vi "4112_Current _Chan Config Dialog_RTM.vi"(8 "error in (no error)":errorcluster, 11 "CD PTR":T1 format="%.0x") -> (0 "error out":errorcluster, 1 "Channels to Add":u16[](array[numeric]), 2 "Voltage Limit (out)":dbl, 3 "Initial Current Value (out)":dbl, 5 "Cancel (out)":bool)   [LabVIEW 2018, in "NI PXI-4110 Programmable Power Supply Custom Device.lvlib"]
doc: "This VI is used to collect all the desired confifugurations for new 4112 Voltage Channels. Note: A true on Sense Mode = Remote and a False = Local."
uses:
  NI PXI-4110 Programmable Power Supply Custom Device.lvlib
  <vilib>/NI Veristand/Custom Device API/Custom Device Item Ref.ctl
  Power_Supply_In_Use.ctl
  4110_Global.vi
  <vilib>/NI Veristand/Custom Device API/Get Item Property (U16).vi
  <vilib>/NI Veristand/Custom Device API/Get Item Property (Boolean).vi
  <vilib>/NI VeriStand/Custom Device API/Custom Device API.lvlib
panel:
  in  "Channel(s) to add":cluster{"Channel 0":bool, "Channel 1":bool}
  in  "Cancel":bool
  in  "OK Button":bool
  in  "Initial Current Value":dbl format="%.4f"
  in  "Voltage Limit":dbl
  # "Current Channels"
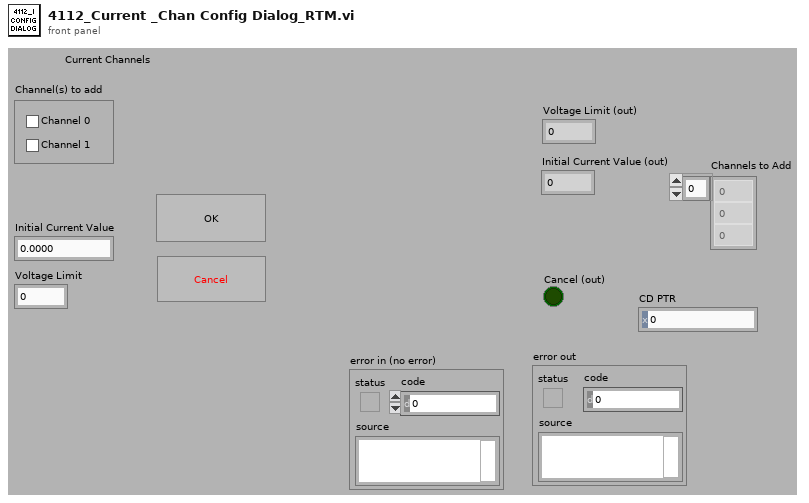
[diagram p1: front panel]
types:
  T1 = typedef "Custom Device API.lvlib/Custom Device Item Ref.ctl" = u64
  T2 = enum8{"Enabled", "Disabled", "Disabled and Grayed Out"}
  T3 = typedef "Custom Device API.lvlib/Custom Device Item Info.ctl" = cluster{"Name":string, "Is Channel":bool, "GUID":string, "Is Waveform":bool}
  T4 = typedef "NI PXI-4110 Programmable Power Supply Custom Device.lvlib/Power_Supply_In_Use.ctl" = enum16{"PXIe-4112", "PXI-4110"}
  T5 = cluster{"V_min":dbl, "V_max":dbl, "I_min":dbl, "I_max":dbl}
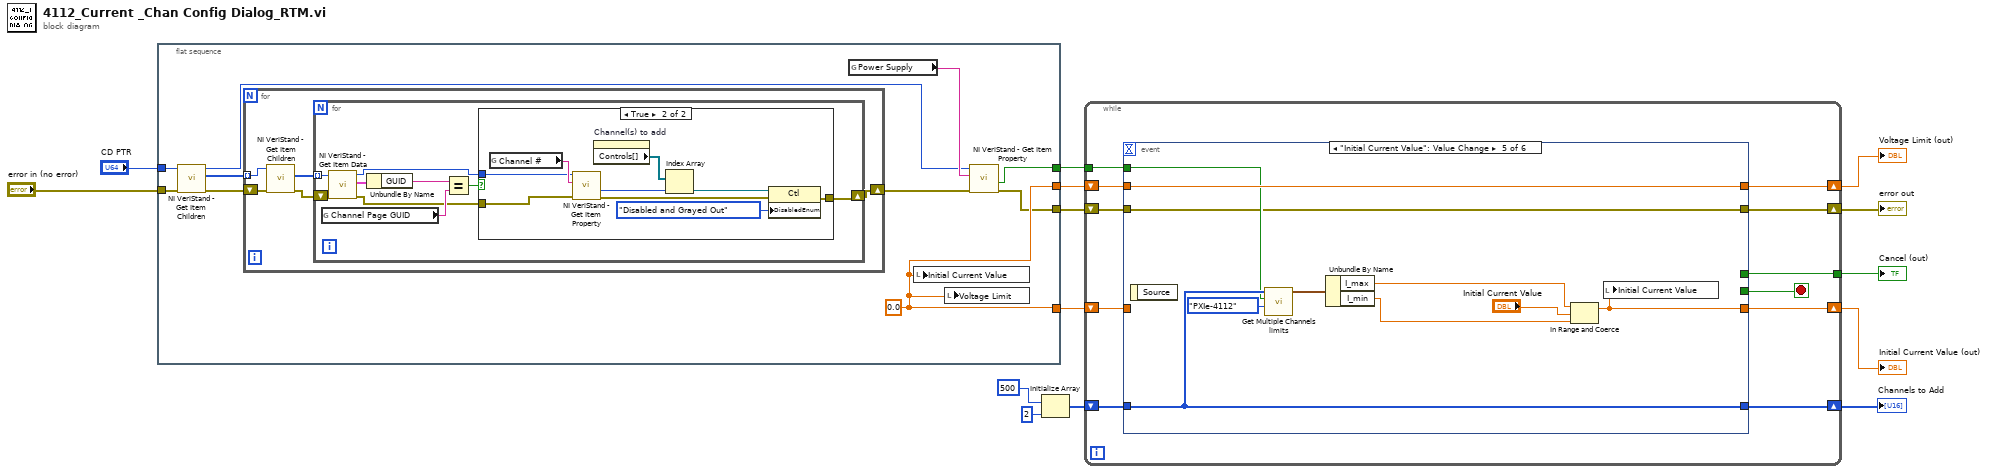
[diagram p0: block diagram]
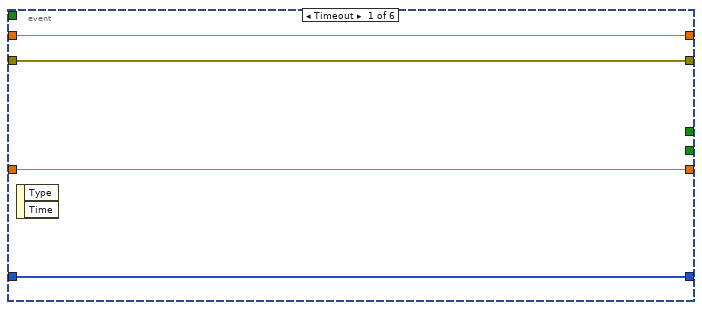
[diagram p3: hidden frame]
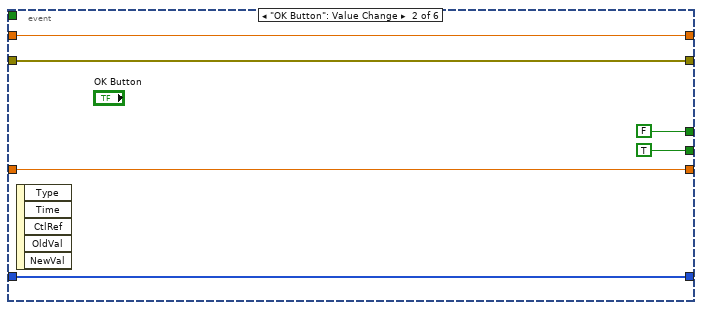
[diagram p4: hidden frame]
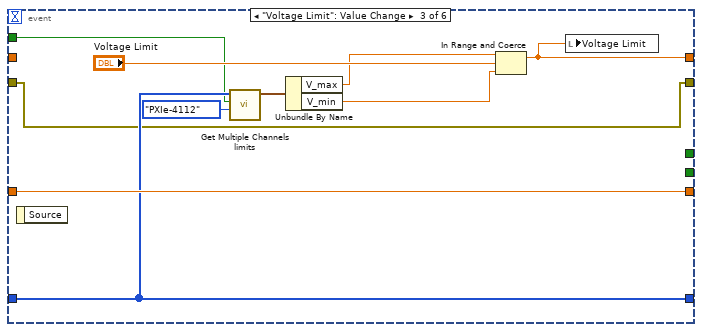
[diagram p5: hidden frame]
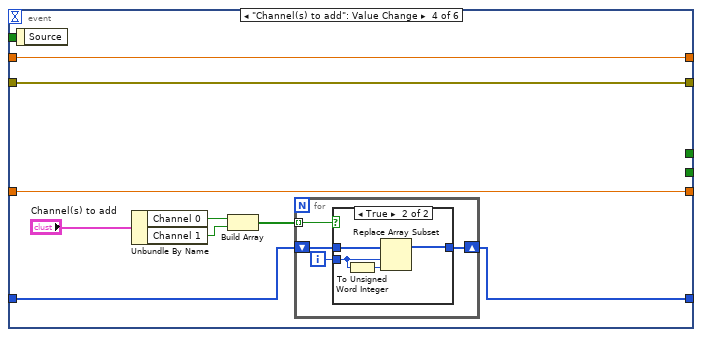
[diagram p6: hidden frame]
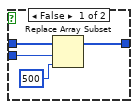
[diagram p7: hidden frame]
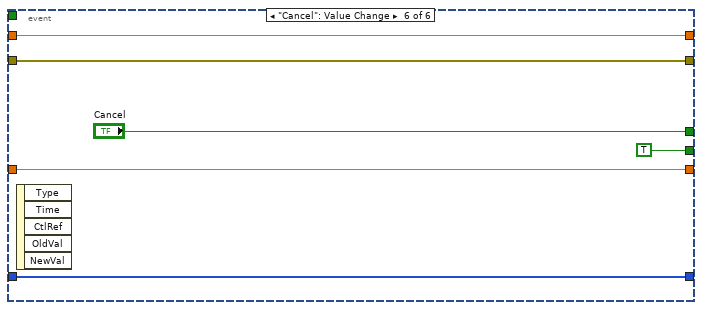
[diagram p8: hidden frame]
diagram:
  n1 = flat-sequence {
    tunnel: [w16] -> w14
    tunnel: [w20] -> w9
    tunnel: [w20] -> w8
    tunnel: "error in (no error)" -> [w24]
    tunnel: "CD PTR" -> [w23]
    tunnel: [w17] -> w5
    frame #0 {
      w20 = 0.0
      n2 = call <vilib>:"NI VeriStand - Get Item Children.vi"("error in (no error)"=w24, "Item Ref in"=w23) -> ("error out"=w21:errorcluster, "Child Refs"=w22:T1[], "Item Ref out"=w15:T1)  [unwired: 6 in, 1 out]
      n3 = for {
        tunnel: w22 -> [w28] mode=indexing
        shift-right: [w29] -> w19
        shift-left: w21 -> [w27]
        n4 = call <vilib>:"NI VeriStand - Get Item Children.vi"("error in (no error)"=w27, "Item Ref in"=w28) -> ("error out"=w25:errorcluster, "Child Refs"=w26:T1[])  [unwired: 6 in, 2 out]
        n5 = for {
          tunnel: w26 -> [w31] mode=indexing
          shift-right: [w38] -> w29
          shift-left: w25 -> [w30]
          n6 = global read "4110_Global.vi" "Channel Page GUID"() -> (w35:string)
          n7 = call <vilib>:"NI VeriStand - Get Item Data.vi"("error in (no error)"=w30, "Item Ref in"=w31) -> ("error out"=w33:errorcluster, "Item Info"=w37:T3, "Item Ref out"=w34:T1)  [unwired: 6 in, 1 out]
          n8 = Unbundle By Name(w37) -> ("GUID"=w36:string)
          n9 = Equal?(x=w36, y=w35) -> (x = y?=w32:bool)
          n10 = case shown="True" w32 {
            tunnel: [w39 w42] -> w38
            tunnel: w34 -> [_ w41]
            tunnel: w33 -> [w39 w40]
            frame False {
            }
            frame True {
              n11 = global read "4110_Global.vi" "Channel #"() -> (w48:string)
              n12 = call-poly <vilib>:"NI VeriStand - Get Item Property.vi"("error in (no error)"=w40, "Property Name"=w48, "Item Ref in"=w41) -> ("error out"=w43:errorcluster, "Value"=w44:u16)  [unwired: 5 in, 2 out]
              n13 = property on="Channel(s) to add" class="Clust (strict)"() -> ("Controls[]"=w46:refnum<vi>[])  [unwired: 2 in, 2 out]
              n14 = Index Array(array=w46, index=w44) -> (element=w47:refnum<vi>)
              n15 = property class="Ctl"(reference=w47, error in=w43, "DisabledEnum"=T2."Disabled and Grayed Out" ("Disabled")) -> (error out=w42:errorcluster)  [unwired: 1 out]
            }
          }
        }
      }
      n16 = global read "4110_Global.vi" "Power Supply"() -> (w18:string)
      n17 = local write "Initial Current Value"(w20) -> ()
      n18 = local write "Voltage Limit"(w20) -> ()
      n19 = call-poly <vilib>:"NI VeriStand - Get Item Property.vi"("error in (no error)"=w19, "Property Name"=w18, "Item Ref in"=w15) -> ("error out"=w16:errorcluster, "Value"=w17:bool)  [unwired: 5 in, 2 out]
    }
  }
  n20 = Initialize Array(u16 500 ("element"), 2 ("dimension size")) -> (w2:u16[])
  n21 = while {
    tunnel: [w55] -> w10
    shift-right: [w58] -> w13
    shift-left: w14 -> [w59]
    shift-right: [w57] -> w12
    shift-left: w9 -> [w53]
    shift-right: [w56] -> w11
    shift-left: w8 -> [w52]
    tunnel: w5 -> [w51]
    shift-right: [w49] -> w1
    shift-left: w2 -> [w50]
    stop <- w54 stop-if-true
    n22 = event shown="[4] \"Initial Current Value\": Value Change" {
      selector: _ -> [_ _ _ _ _ _]
      dyn-events: _ -> [_ _ _ _ _ _]
      timeout: _ -> [_ _ _ _ _ _]
      tunnel: [w63 w66 w79 w88 w109 w114] -> w57
      tunnel: [w62 w65 w77 w87 w108 w113] -> w56
      tunnel: w59 -> [w60 w69 w70 w80 w101 w111]
      tunnel: [w60 w69 w70 w80 w101 w111] -> w58
      tunnel: [_ FALSE ("Cancel") _ _ _ "Cancel"] -> w55
      tunnel: [_ TRUE ("Cancel") _ _ _ TRUE ("Cancel")] -> w54
      tunnel: w53 -> [w63 w66 w79 w88 _ w114]
      tunnel: w52 -> [w62 w65 _ w87 w108 w113]
      tunnel: w51 -> [_ _ w75 _ w106 _]
      tunnel: w50 -> [w61 w64 w76 w82 w107 w112]
      tunnel: [w61 w64 w76 w81 w107 w112] -> w49
      event Timeout {
        n23 = event-data() -> ()  [unwired: 1 in, 2 out]
      }
      event "OK Button": Value Change {
        n24 = event-data() -> ()  [unwired: 1 in, 5 out]
      }
      event "Voltage Limit": Value Change {
        n25 = event-data() -> ()  [unwired: 1 in, 1 out]
        n26 = call "Get Multiple Channels limits.vi"("Power Supply In Use"=Power_Supply_In_Use."PXIe-4112", "External Supply?"=w75, "Channels"=w76) -> ("output cluster"=w73:T5)  [unwired: 7 in, 1 out]
        n27 = Unbundle By Name(w73) -> ("V_max"=w72:dbl, "V_min"=w71:dbl)
        n28 = In Range and Coerce(upper limit=w72, x="Voltage Limit", lower limit=w71) -> (coerced(x)=w77:dbl)  [unwired: 1 out]
        n29 = local write "Voltage Limit"(w77) -> ()
      }
      event "Channel(s) to add": Value Change {
        n30 = event-data() -> ()  [unwired: 1 in, 1 out]
        n31 = Unbundle By Name("Channel(s) to add") -> ("Channel 0"=w85:bool, "Channel 1"=w84:bool)
        n32 = Build Array(w85, w84) -> (w83:bool[])
        n33 = for {
          tunnel: w83 -> [w92] mode=indexing
          shift-right: [w89] -> w81
          shift-left: w82 -> [w91]
          i -> [w90]
          n34 = case shown="True" w92 {
            tunnel: w91 -> [w95 w100]
            tunnel: w90 -> [w96 w98]
            tunnel: [w93 w99] -> w89
            frame False {
              n35 = Replace Array Subset(array=w95, new element=u16 500 ("new element/subarray"), index=w96) -> (w93:u16[])
            }
            frame True {
              n36 = To Unsigned Word Integer(number=w98) -> (unsigned 16bit integer=w97:u16)
              n37 = Replace Array Subset(array=w100, new element=w97, index=w98) -> (w99:u16[])
            }
          }
        }
      }
      event "Initial Current Value": Value Change {
        n38 = event-data() -> ()  [unwired: 1 in, 1 out]
        n39 = call "Get Multiple Channels limits.vi"("Power Supply In Use"=Power_Supply_In_Use."PXIe-4112", "External Supply?"=w106, "Channels"=w107) -> ("output cluster"=w104:T5)  [unwired: 7 in, 1 out]
        n40 = Unbundle By Name(w104) -> ("I_max"=w103:dbl, "I_min"=w102:dbl)
        n41 = In Range and Coerce(upper limit=w103, x="Initial Current Value", lower limit=w102) -> (coerced(x)=w109:dbl)  [unwired: 1 out]
        n42 = local write "Initial Current Value"(w109) -> ()
      }
      event "Cancel": Value Change {
        n43 = event-data() -> ()  [unwired: 1 in, 5 out]
      }
    }
  }
  "error out" <- w13
  "Initial Current Value (out)" <- w12
  "Voltage Limit (out)" <- w11
  "Cancel (out)" <- w10
  "Channels to Add" <- w1
